vi "Run Step Async.vi"(8 "error in (no error)":errorcluster, 10 "Step in":refnum<class "Step.lvclass">, 11 "Tester in":refnum<class "Tester.lvclass">) -> (0 "error out":errorcluster, 2 "Step out":refnum<class "Step.lvclass">)   [LabVIEW 2020, in "Tester.lvlib" / "Tester.lvclass"]
uses:
  Tester.lvclass
  Step/Step.lvclass
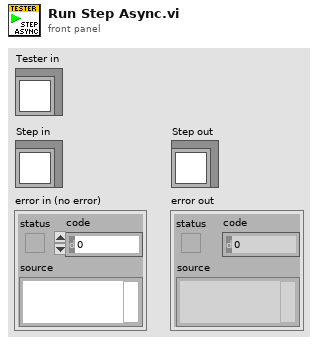
[diagram p1: front panel]
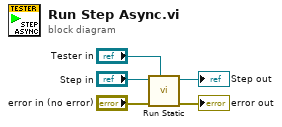
[diagram p0: block diagram]
diagram:
  n1 = call "Run Static.vi"("Tester"="Tester in", "error in (no error)"="error in (no error)", "Step in"="Step in") -> ("error out"=→"error out":errorcluster, "Step out"=→"Step out":refnum<class "Step.lvclass">)  [unwired: 7 in]
